vi "Create Rooms List Map.vi"(11 "error in (no error)":errorcluster) -> (4 "Rooms List Map":map{string, T1}(c390), 15 "error out":errorcluster)   [LabVIEW 2023, in "File Data Manager.lvlib" / "File Data Manager.lvclass"]
uses:
  File Data Manager.lvclass
  Central Data Manager/Central Data Manager/Room Details.ctl
  Central Data Manager/Central Data Manager/Room Occupancy Status.ctl
  Central Data Manager/Central Data Manager/Guest Details.ctl
  6d55522a-4221-4587-be62-d131c33c8ae9.vi
  <vilib>/Utility/file.llb/Read Delimited Spreadsheet (string).vi
  File Data Manager.lvclass/File Data Manager.ctl
  Utilities/Utilities.lvlib
  Central Data Manager/Central Data Manager/Central Data Manager.lvclass
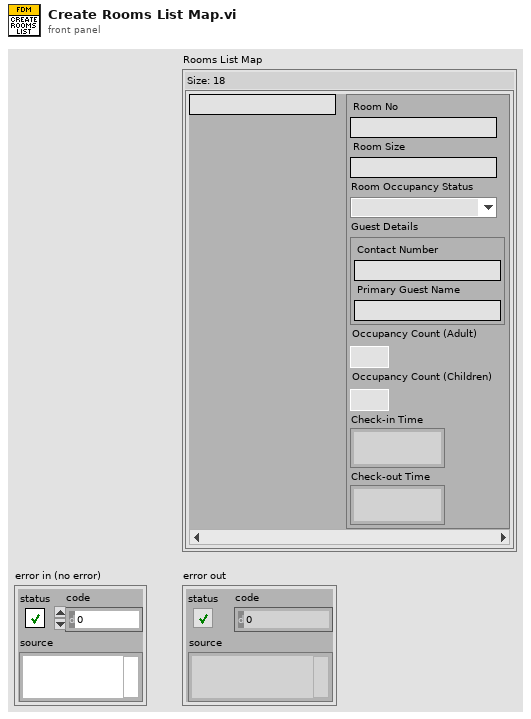
[diagram p1: front panel]
types:
  T1 = typedef "Central Data Manager.lvlib/Central Data Manager.lvclass/Room Details.ctl" = cluster{"Room No":string, "Room Size":string, "Room Occupancy Status":T2, "Guest Details":T3, "Occupancy Count (Adult)":u32, "Occupancy Count (Children)":u32, "Check-in Time":timestamp, "Check-out Time":timestamp}
  T2 = typedef "Central Data Manager.lvlib/Central Data Manager.lvclass/Room Occupancy Status.ctl" = enum16{"Not Occupied", "Occupied", "Under Maintainance", "Not Servicable"}
  T3 = typedef "Central Data Manager.lvlib/Central Data Manager.lvclass/Guest Details.ctl" = cluster{"Contact Number":string, "Primary Guest Name":string}
  T4 = typedef "Hotel Management Tool Model.lvlib/Hotel Management Tool Model.lvclass/Database File Paths.ctl" = cluster{"Food Menu File Path":path, "Guests Histroy File Path":path, "Room Size File Path":path, "Rooms List File Path":path, "Rooms Service Allocation File Path":path, "Staff List File Path":path}
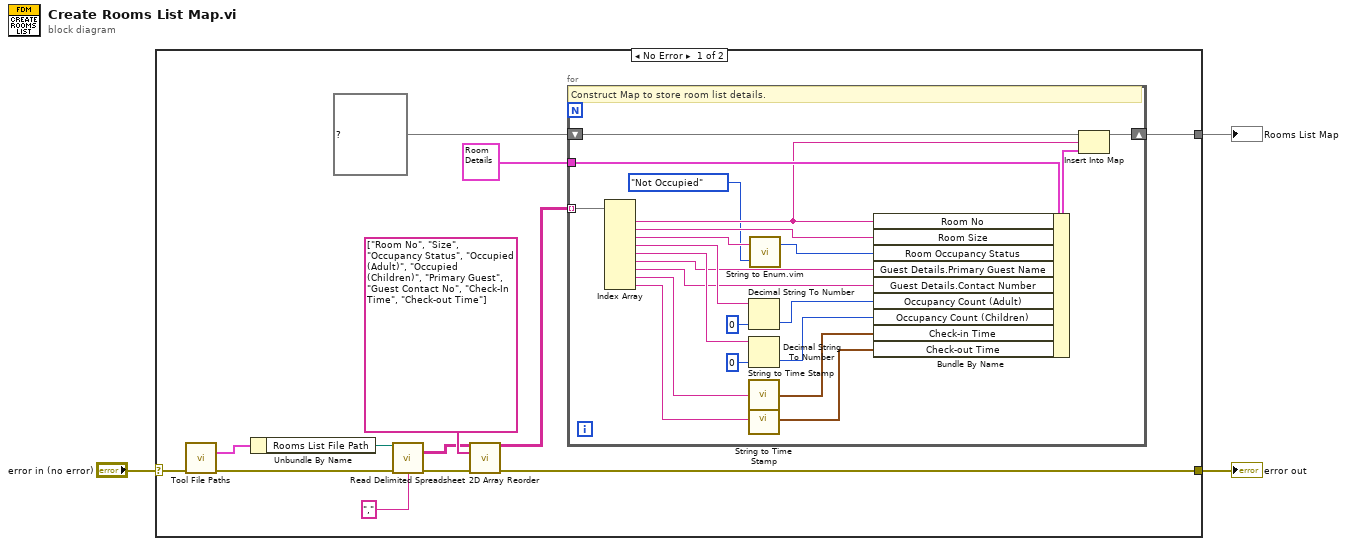
[diagram p0: block diagram]
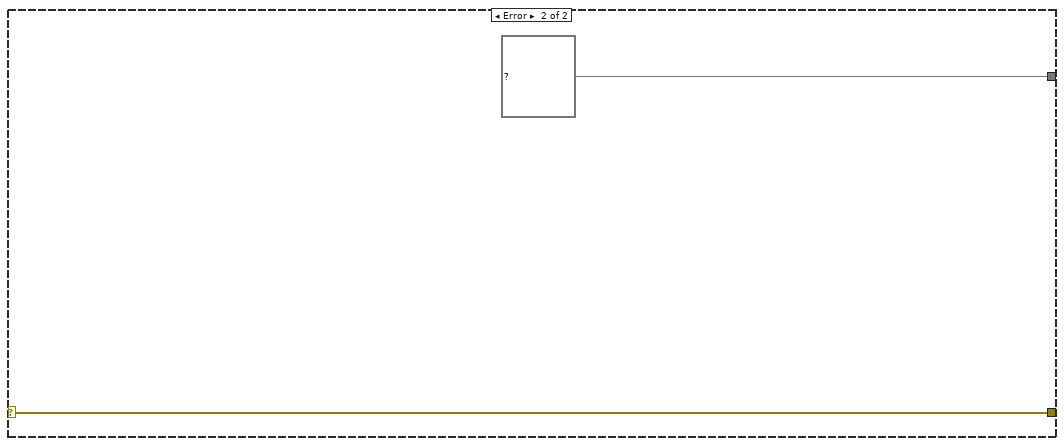
[diagram p2: hidden frame]
diagram:
  n1 = case shown="No Error" "error in (no error)" {
    selector: "error in (no error)" -> [w9 w40]
    tunnel: [w5 w40] -> w2
    tunnel: [w4 map{string, T1} {} ("Rooms List")] -> w1
    frame No Error {
      n2 = call "Tool File Paths.vi"("error in (no error)"=w9) -> ("Database File Paths"=w16:T4, "error out"=w15:errorcluster)  [unwired: 12 in, 1 out]
      n3 = Unbundle By Name(w16) -> ("Rooms List File Path"=w14:path)
      n4 = call-poly <vilib>:"Read Delimited Spreadsheet.vi"("file path (dialog if empty)"=w14, "error in (no error)"=w15, "delimiter (\\t)"="," ("delimiter (\\t)")) -> ("all rows"=w10:string[][], "error out"=w11:errorcluster)  [unwired: 7 in, 4 out]
      n5 = call "2D Array Reorder.vi"("2D Array Data witjh Header"=w10, "Header Order"=string[] ["Room No", "Size", "Occupancy Status", "Occupied (Adult)", "Occupied (Children)", "Primary Guest", "Guest Contact No", "Check-In Time", "Check-out Time"] ("first row"), "error in (no error)"=w11) -> ("Reordered Data without Header"=w6:string[][], "error out"=w5:errorcluster)  [unwired: 11 in]
      n6 = for {
        tunnel: w6 -> [w35] mode=indexing
        shift-right: [w37] -> w4
        shift-left: map{string, T1} {} ("Rooms List") -> [w38]
        tunnel: T1 {"Room No"="", "Room Size"="", "Room Occupancy Status"=enum."Not Occupied", "Guest Details"={"Contact Number"="", "Primary Guest Name"=""}, "Occupancy Count (Adult)"=0, "Occupancy Count (Children)"=0, "Check-in Time"=timestamp(0 s since 1904-01-01), "Check-out Time"=timestamp(0 s since 1904-01-01)} ("Room Details") -> [w36]
        # "Construct Map to store room list details."
        n7 = Index Array(array=w35) -> (element #1=w34:string, element #2=w28:string, element #3=w19:string, element #4=w27:string, element #5=w26:string, element #6=w25:string, element #7=w24:string, element #8=w23:string, element #9=w22:string)  [unwired: 9 in]
        n8 = Decimal String To Number(string=w27, default (0L)=u32 0 ("Cost Per Day (Rs)")) -> (number=w30:u32)  [unwired: 1 in, 1 out]
        n9 = Decimal String To Number(string=w26, default (0L)=u32 0 ("Cost Per Day (Rs)")) -> (number=w29:u32)  [unwired: 1 in, 1 out]
        n10 = call "String to Time Stamp.vi"("input string"=w23) -> ("output 1"=w21:timestamp)
        n11 = call "String to Time Stamp.vi"("input string"=w22) -> ("output 1"=w20:timestamp)
        n12 = call "String to Enum.vim"("Enum Type"=Room_Occupancy_Status."Not Occupied" ("Room Occupancy Status"), "Input String"=w19) -> ("Output"=w18:T2)
        n13 = Bundle By Name(cluster=w36, "Room No"=w34, "Room Size"=w28, "Room Occupancy Status"=w18, "Guest Details.Primary Guest Name"=w25, "Guest Details.Contact Number"=w24, "Occupancy Count (Adult)"=w30, "Occupancy Count (Children)"=w29, "Check-in Time"=w21, "Check-out Time"=w20) -> (w31:T1)
        n14 = Insert Into Map(map in=w38, key=w34, value=w31) -> (map out=w37:map{string, T1})  [unwired: 2 out]
      }
    }
    frame Error {
    }
  }
  "error out" <- w2
  "Rooms List Map" <- w1
